vi "XIPIN_Image_Noise_Reduction_5_01_a.vi"   [LabVIEW 2017]
doc: "The Xilinx Noise Reduction LogiCORE provides developers with an easy to use IP block for reducing noise within each frame of video. The core has a programmable, edge adaptive smoothing function to change the characteristics of the filtering in real-time.\n------------------------------------\n<b>Need License</b> : Yes\n<b>Interface</b> : AXI4-Stream AXI4-Lite"
uses:
  <vilib>/rvi/XilinxIP/XIPIN_XNode/niFpgaXIPIN.xnode
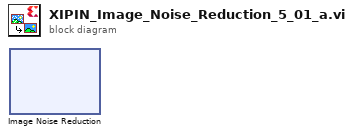
[diagram p0: block diagram]
diagram:
  n1 = xnode ("Image Noise Reduction")() -> ()
